vi "Intake Command Helper.vi"(7 "Description":string, 8 "Command Info In":T3, 11 "SubSystem Data":T1) -> (0 "Command Info Out":T3, 1 "Command Timing":cluster{"Start Time (ms)":u32, "Iterations":i32}, 3 "SubSystem Data":T1)   [LabVIEW 2017]
uses:
  Intake Setpoints.ctl
  Intake Operations.ctl
  <vilib>/Rock Robotics/WPI/Framework/Command Status Info.ctl
  <vilib>/Rock Robotics/WPI/Framework/Completion Status.ctl
  <vilib>/Rock Robotics/WPI/Framework/Completion Notifier.ctl
  Framework/Robot Global Data.vi
  Intake Published Globals.vi
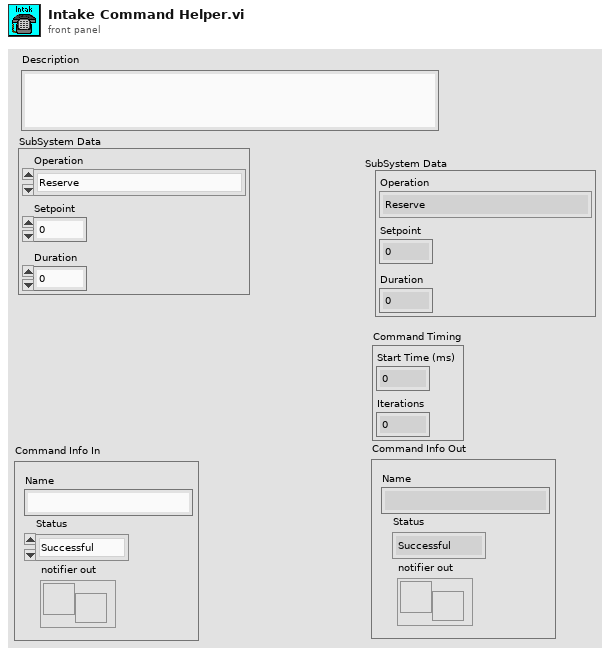
[diagram p1: front panel]
types:
  T1 = typedef "Intake Setpoints.ctl" = cluster{"Operation":T2, "Setpoint":dbl, "Duration":dbl}
  T2 = typedef "Intake Operations.ctl" = enum16{"Reserve", "Read Current", "Immediate", "Intake", "Eject", "Stop"}
  T3 = typedef "Command Status Info.ctl" = cluster{"Name":string, "Status":T4, "notifier out":T5}
  T4 = typedef "Completion Status.ctl" = enum16{"Successful", "Aborted", "Incomplete"}
  T5 = typedef "Completion Notifier.ctl" = refnum<notifier>
  T6 = cluster{"Current Command":T1, "Command Timing":cluster{"Start Time (ms)":u32, "Iterations":i32}, "Command Arguments":cluster{"Command Info":T3, "Description":string, "Default Command":T1, "queue out":refnum<queue>, "Subsystem Name":string}}
  T7 = cluster{"SubSystem Data":T1, "Command Info In":T3, string}
  T8 = cluster{"Command Info":T3, "Description":string, "Default Command":T1, "queue out":refnum<queue>, "Subsystem Name":string}
  T9 = cluster{"SubSystem Data":T1, "Command Info In":T3, "Description":string}
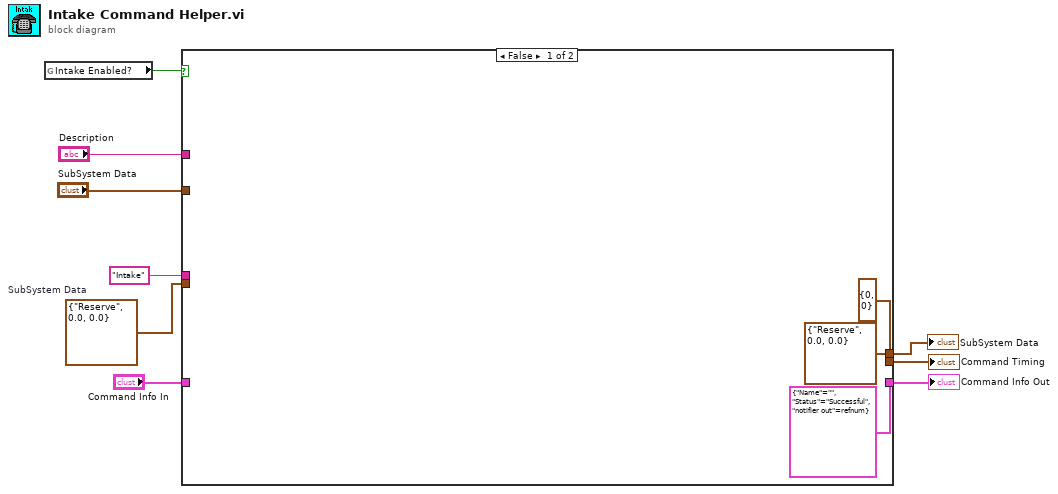
[diagram p0: block diagram]
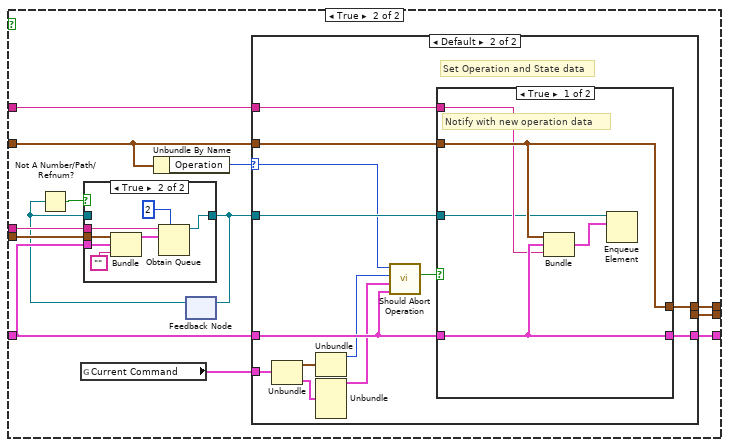
[diagram p2: hidden frame]
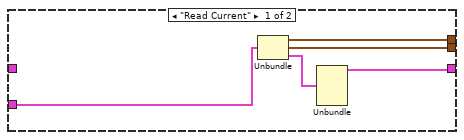
[diagram p4: hidden frame]
diagram:
  w5 = T1 {"Operation"=enum."Reserve", "Setpoint"=0.0, "Duration"=0.0}  # SubSystem Data
  n1 = global read "Robot Global Data.vi" "Intake Enabled?"() -> (w1:bool)
  n2 = case shown="False" w1 {
    tunnel: "SubSystem Data" -> [_ w25]
    tunnel: "Intake" -> [_ w23]
    tunnel: [T3 {"Name"="", "Status"=enum."Successful", "notifier out"=refnum} ("Command Info In") w21] -> w7
    tunnel: "Command Info In" -> [_ w20]
    tunnel: w5 -> [_ w19]
    tunnel: [T1 {"Operation"=enum."Reserve", "Setpoint"=0.0, "Duration"=0.0} ("SubSystem Data") w18] -> w4
    tunnel: "Description" -> [_ w15]
    tunnel: [cluster{"Start Time (ms)":u32, "Iterations":i32} {"Start Time (ms)"=0, "Iterations"=0} ("Command Timing") w14] -> w2
    frame False {
    }
    frame True {
      n3 = global read "Intake Published Globals.vi" "Current Command"() -> (w13:T6)
      n4 = Unbundle By Name(w25) -> ("Operation"=w24:T2)
      n5 = feedback #1() -> (w16:refnum<queue>)  [unwired: 1 in]
      n6 = Not A Number/Path/Refnum?(number/path/refnum=w16) -> (NaN/Path/Refnum?=w17:bool)
      n7 = case shown="True" w17 {
        tunnel: w23 -> [_ w30]
        tunnel: [w26 w28] -> w22
        tunnel: w19 -> [_ w33]
        tunnel: w20 -> [_ w32]
        tunnel: w16 -> [w26 _]
        frame False {
        }
        frame True {
          n8 = Bundle("SubSystem Data"=w33, "Command Info In"=w32, "") -> (w29:T7)  [unwired: 1 in]
          n9 = Obtain Queue(max queue size (-1, unlimited)=2, name (unnamed)=w30, element data type=w29) -> (queue out=w28:refnum<queue>)  [unwired: 2 in, 2 out]
        }
      }
      n10 = feedback-in #1(w22) -> ()
      n11 = case shown="Default" w24 {
        selector: w24 -> [_ w46]
        tunnel: [w37 w48] -> w18
        tunnel: w22 -> [_ w50]
        tunnel: w25 -> [_ w51]
        tunnel: [w36 w49] -> w21
        tunnel: w20 -> [_ w45]
        tunnel: w15 -> [_ w44]
        tunnel: [w35 _] -> w14
        tunnel: w13 -> [w34 w43]
        frame "Read Current" {
          n12 = Unbundle(w34) -> ("Current Command"=w37:T1, "Command Timing"=w35:cluster{"Start Time (ms)":u32, "Iterations":i32}, "Command Arguments"=w38:T8)
          n13 = Unbundle(w38) -> ("Command Info"=w36:T3)  [unwired: 4 out]
        }
        frame Default {
          # "Set Operation and State data"
          n14 = Unbundle(w43) -> ("Current Command"=w42:T1, "Command Arguments"=w40:T8)  [unwired: 1 out]
          n15 = Unbundle(w42) -> ("Operation"=w41:T2)  [unwired: 2 out]
          n16 = Unbundle(w40) -> ("Command Info"=w39:T3)  [unwired: 4 out]
          n17 = call <vilib>:"Should Abort Operation.vi"("New Command Info"=w45, "Command Info"=w39, "Current Operation"=w41, "New Operation"=w46) -> ("Execute"=w47:bool)  [unwired: 7 in]
          n18 = case shown="True" w47 {
            tunnel: [w56 _] -> w48
            tunnel: w51 -> [w56 _]
            tunnel: w50 -> [w53 _]
            tunnel: [w55 w57] -> w49
            tunnel: w45 -> [w55 w57]
            tunnel: w44 -> [w54 _]
            frame True {
              # "Notify with new operation data"
              n19 = Bundle("SubSystem Data"=w56, "Command Info In"=w55, "Description"=w54) -> (w52:T9)  [unwired: 1 in]
              n20 = Enqueue Element(queue=w53, element=w52) -> ()  [unwired: 2 in, 3 out]
            }
            frame False {
              # "This operation will not be\nexecuted. Upstream command\nwas aborted."
            }
          }
        }
      }
    }
  }
  "Command Info Out" <- w7
  "SubSystem Data" <- w4
  "Command Timing" <- w2
